vi "ADCP_Open_Node_Connection.vi"(8 "error in (no error)":errorcluster, 10 "Node ID":i32=-1, 11 "ADCP In":refnum<class "ADCP.lvclass">) -> (0 "error out":errorcluster, 3 "ADCP Out":refnum<class "ADCP.lvclass">)   [LabVIEW 2017, in "ADCP.lvclass"]
uses:
  ADCP.lvclass
  ADCP.lvclass/ADCP.ctl
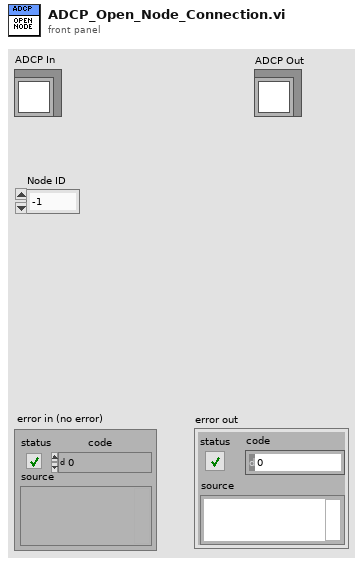
[diagram p1: front panel]
types:
  T1 = cluster{"CC_ACK":bool, "CC_RQST":bool, "OC_ACK":bool, "OC_RQST":bool, "SYNC_ACK":bool, "SYNC_RQST":bool}
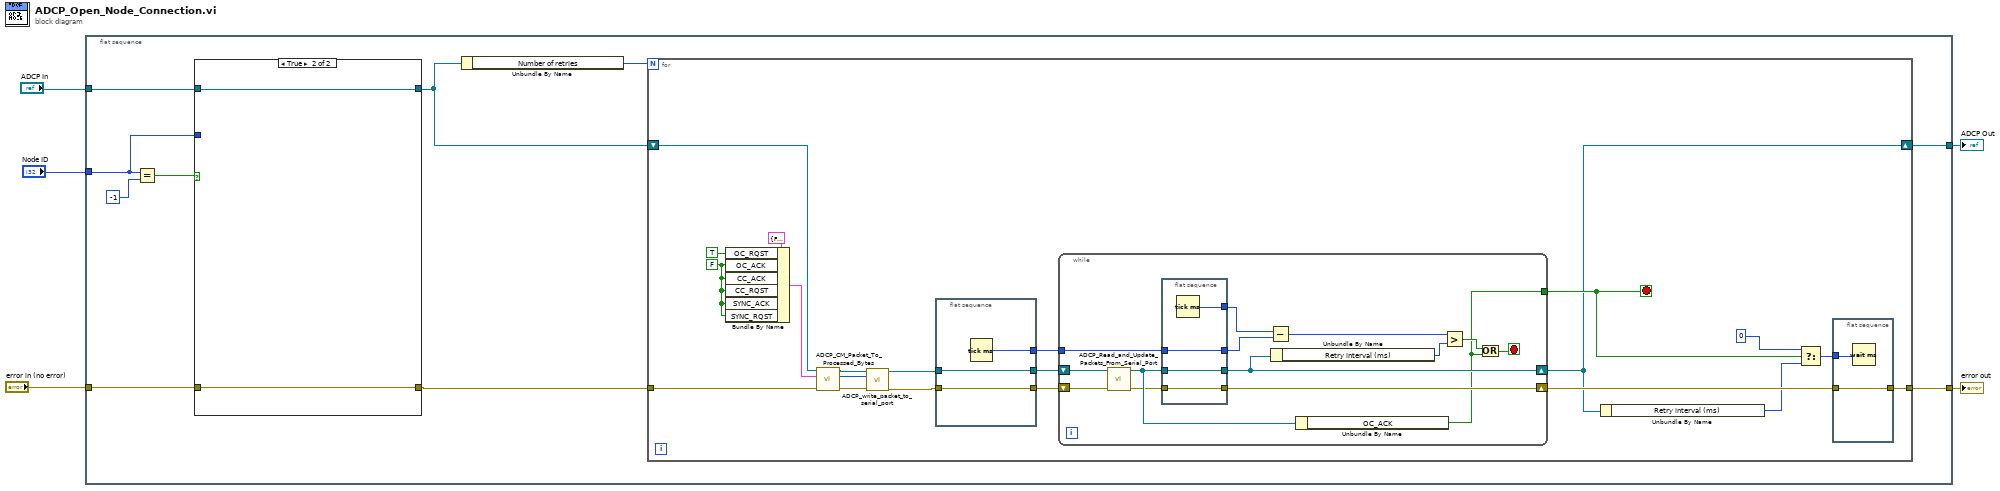
[diagram p0: block diagram]
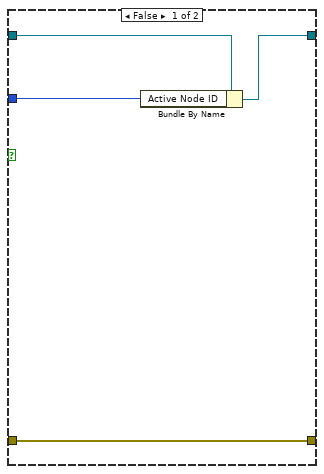
[diagram p2: hidden frame]
diagram:
  n1 = flat-sequence {
    tunnel: "ADCP In" -> [w12]
    tunnel: "error in (no error)" -> [w14]
    tunnel: "Node ID" -> [w11]
    tunnel: [w7] -> w2
    tunnel: [w6] -> w1
    frame #0 {
      n2 = Equal?(x=w11, y=-1) -> (x = y?=w13:bool)
      n3 = case shown="True" w13 {
        tunnel: w14 -> [w60 w64]
        tunnel: w12 -> [w63 w65]
        tunnel: [w61 w65] -> w8
        tunnel: w11 -> [w62 _]
        tunnel: [w60 w64] -> w10
        frame False {
          n4 = Bundle By Name(cluster=w63, "Active Node ID"=w62) -> (w61:refnum<class "ADCP.lvclass">)
        }
        frame True {
        }
      }
      n5 = Unbundle By Name(w8) -> ("Number of retries"=w9:u16)
      n6 = for {
        N: w9 -> [_]
        tunnel: w10 -> [w36]
        shift-right: [w23] -> w7
        shift-left: w8 -> [w35]
        tunnel: [w21] -> w6
        stop <- w26 stop-if-true
        w31 = FALSE ("OC_ACK")
        n7 = Bundle By Name(cluster=T1 {"CC_ACK"=FALSE, "CC_RQST"=FALSE, "OC_ACK"=FALSE, "OC_RQST"=FALSE, "SYNC_ACK"=FALSE, "SYNC_RQST"=FALSE} ("ADCP Connection Management Packet"), "OC_RQST"=TRUE ("OC_ACK"), "OC_ACK"=w31, "CC_ACK"=w31, "CC_RQST"=w31, "SYNC_ACK"=w31, "SYNC_RQST"=w31) -> (w32:T1)
        n8 = call "ADCP_CM_Packet_To_Processed_Bytes.vi"("error in (no error)"=w36, "Connection Management"=w32, "ADCP in"=w35) -> ("error out"=w18:errorcluster, "Processed Packet"=w20:u8[], "ADCP out"=w19:refnum<class "ADCP.lvclass">)  [unwired: 6 in]
        n9 = call "ADCP_write_packet_to_serial_port.vi"("error in (no error)"=w18, "Packet Bytes"=w20, "ADCP In"=w19) -> ("error out"=w17:errorcluster, "ADCP Out"=w16:refnum<class "ADCP.lvclass">)  [unwired: 7 in]
        n10 = flat-sequence {
          tunnel: w16 -> [w41]
          tunnel: [w41] -> w30
          tunnel: w17 -> [w40]
          tunnel: [w40] -> w29
          tunnel: [w39] -> w28
          frame #0 {
            n11 = Tick Count (ms)() -> (millisecond timer value=w39:u32)
          }
        }
        n12 = while {
          shift-right: [w46] -> w23
          shift-left: w30 -> [w54]
          shift-right: [w51] -> w27
          shift-left: w29 -> [w55]
          tunnel: w28 -> [w49]
          tunnel: [w42] -> w26
          stop <- w43 stop-if-true
          n13 = call "ADCP_Read_and_Update_Packets_From_Serial_Port.vi"("error in (no error)"=w55, "ADCP In"=w54) -> ("error out"=w52:errorcluster, "ADCP out"=w53:refnum<class "ADCP.lvclass">)  [unwired: 6 in, 2 out]
          n14 = flat-sequence {
            tunnel: w53 -> [w59]
            tunnel: [w59] -> w46
            tunnel: w52 -> [w58]
            tunnel: [w58] -> w51
            tunnel: [w57] -> w50
            tunnel: w49 -> [w56]
            tunnel: [w56] -> w48
            frame #0 {
              n15 = Tick Count (ms)() -> (millisecond timer value=w57:u32)
            }
          }
          n16 = Subtract(x=w50, y=w48) -> (x-y=w47:u32)
          n17 = Unbundle By Name(w46) -> ("Retry interval (ms)"=w45:u16)
          n18 = Unbundle By Name(w53) -> ("OC_ACK"=w42:bool)
          n19 = Greater?(x=w47, y=w45) -> (0:w44:bool)
          n20 = Or(x=w44, y=w42) -> (x .or. y?=w43:bool)
        }
        n21 = Unbundle By Name(w23) -> ("Retry interval (ms)"=w22:u16)
        n22 = Select(t=0, s=w26, f=w22) -> (s? t:f=w24:i32)
        n23 = flat-sequence {
          tunnel: w27 -> [w38]
          tunnel: [w38] -> w21
          tunnel: w24 -> [w37]
          frame #0 {
            n24 = Wait (ms)(milliseconds to wait=w37) -> ()  [unwired: 1 out]
          }
        }
      }
    }
  }
  "ADCP Out" <- w2
  "error out" <- w1
